vi "create Connect.vi"(8 "error in (no error)":errorcluster, 11 "Connect in":refnum<class "Connect.lvclass">) -> (0 "error out":errorcluster, 3 "Connect out":refnum<class "Connect.lvclass">)   [LabVIEW 2019, in "Connect.lvclass"]
uses:
  Connect.lvclass
  TCP Packet/Packet.lvclass
  TCP Packet/packet type STYP.ctl
  C:/projects/labview_multiplayer_snake/Main Codeline/Software/Code/Shared/TCP Packet/Packet.lvclass
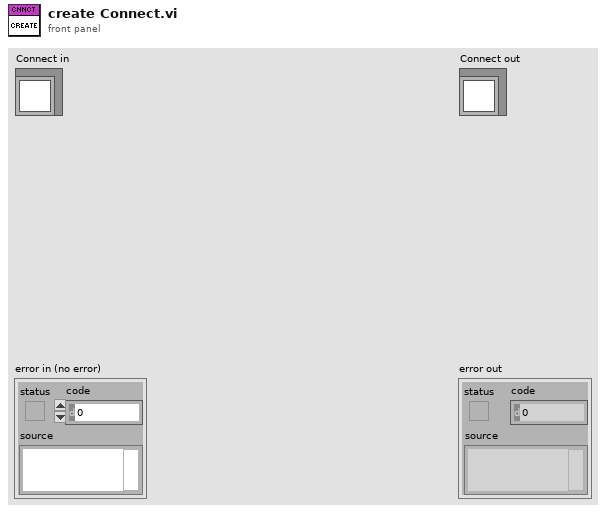
[diagram p1: front panel]
types:
  T1 = typedef "Packet.lvclass/packet type STYP.ctl" = enum16{"Connect", "Disconnect", "Direction", "Score", "Map"}
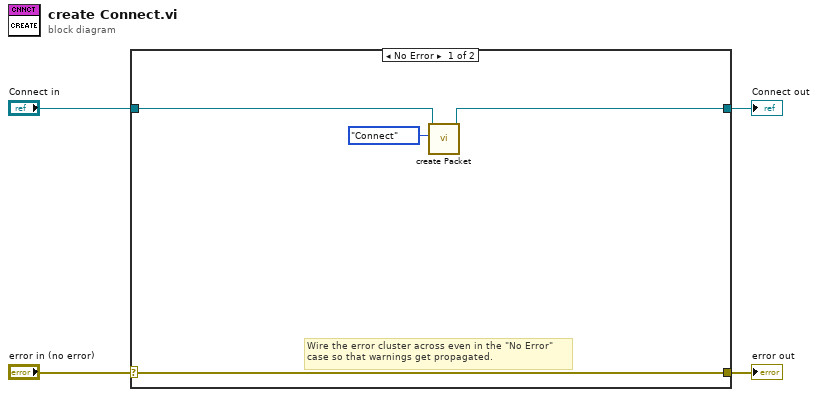
[diagram p0: block diagram]
diagram:
  n1 = case shown="No Error" "error in (no error)" {
    selector: "error in (no error)" -> [w8 w10]
    tunnel: [w8 w10] -> w3
    tunnel: [w7 w9] -> w1
    tunnel: "Connect in" -> [w6 w9]
    frame No Error {
      # "Wire the error cluster across even in the \"No Error\"\ncase so that warnings get propagated."
      n2 = call "create Packet.vi"("Packet Type"=packet_type_STYP."Connect", "Packet in"=w6) -> ("Packet out"=w7:refnum<class "Connect.lvclass">)  [unwired: 8 in, 1 out]
    }
    frame Error {
    }
  }
  "error out" <- w3
  "Connect out" <- w1
